vi "GetRollingAverage.vi"(8 "Error In":errorcluster, 10 "Datum":dbl, 11 "Rolling Average Queue In":refnum<queue>) -> (0 "Error Out":errorcluster, 1 "Non-Zero Rolling Average":dbl, 2 "Rolling Average":dbl format="%0.2f", 3 "Rolling Average Queue Out":refnum<queue>)   [LabVIEW 2012, in "LV-Utilities.lvlib"]
uses:
  LV-Utilities.lvlib
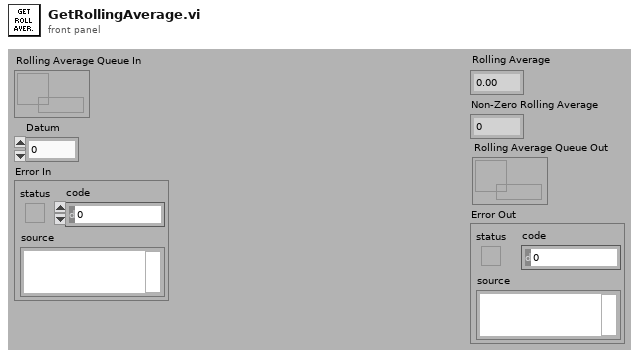
[diagram p1: front panel]
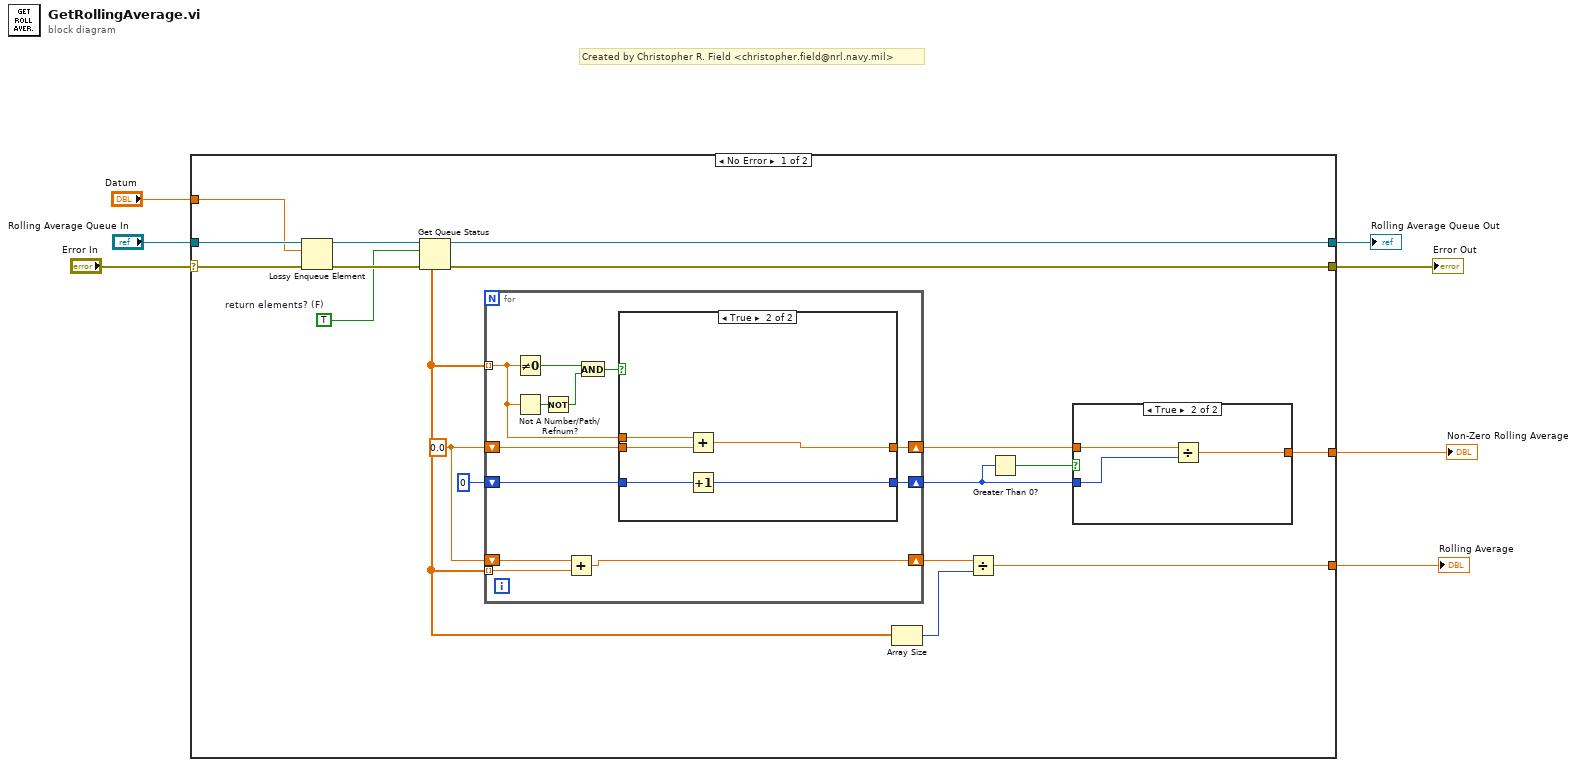
[diagram p0: block diagram]
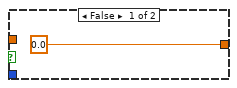
[diagram p2: hidden frame]
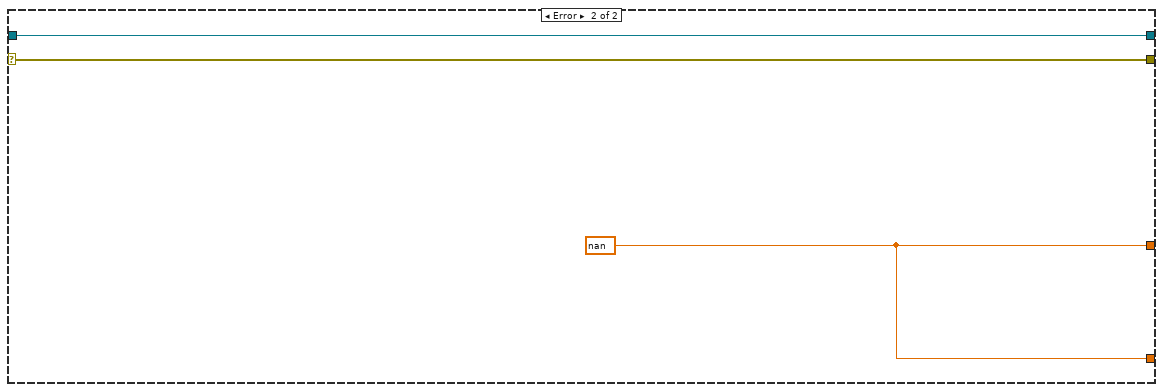
[diagram p4: hidden frame]
diagram:
  # "Created by Christopher R. Field <christopher.field@nrl.navy.mil>"
  n1 = case shown="No Error" "Error In" {
    selector: "Error In" -> [w8 w50]
    tunnel: "Rolling Average Queue In" -> [w25 w51]
    tunnel: "Datum" -> [w24 _]
    tunnel: [w18 w49] -> w5
    tunnel: [w17 w51] -> w4
    tunnel: [w16 w50] -> w3
    tunnel: [w9 w49] -> w2
    frame No Error {
      w13 = 0.0
      w21 = TRUE  # return elements? (F)
      n2 = Lossy Enqueue Element(queue=w25, element=w24, error in (no error)=w8) -> (queue out=w23:refnum<queue>, error out=w22:errorcluster)  [unwired: 2 out]
      n3 = Get Queue Status(queue=w23, return elements? (F)=w21, error in (no error)=w22) -> (queue out=w17:refnum<queue>, error out=w16:errorcluster, elements=w12:dbl[])  [unwired: 5 out]
      n4 = for {
        tunnel: w12 -> [w34] mode=indexing
        shift-right: [w38] -> w19
        shift-left: w13 -> [w41]
        shift-right: [w39] -> w15
        shift-left: 0 -> [w40]
        tunnel: w12 -> [w36] mode=indexing
        shift-right: [w35] -> w11
        shift-left: w13 -> [w37]
        n5 = Not Equal To 0?(x=w34) -> (x != 0?=w32:bool)
        n6 = Not A Number/Path/Refnum?(number/path/refnum=w34) -> (NaN/Path/Refnum?=w33:bool)
        n7 = Not(x=w33) -> (.not. x?=w31:bool)
        n8 = Add(x=w37, y=w36) -> (x+y=w35:dbl)
        n9 = And(x=w32, y=w31) -> (x .and. y?=w30:bool)
        n10 = case shown="True" w30 {
          tunnel: w34 -> [_ w48]
          tunnel: w41 -> [w43 w47]
          tunnel: w40 -> [w42 w46]
          tunnel: [w42 w45] -> w39
          tunnel: [w43 w44] -> w38
          frame False {
          }
          frame True {
            n11 = Add(x=w48, y=w47) -> (x+y=w44:dbl)
            n12 = Increment(x=w46) -> (x+1=w45:i32)
          }
        }
      }
      n13 = Array Size(array=w12) -> (size(s)=w10:i32)
      n14 = Divide(x=w11, y=w10) -> (x/y=w9:dbl)
      n15 = Greater Than 0?(x=w15) -> (x > 0?=w14:bool)
      n16 = case shown="True" w14 {
        tunnel: w19 -> [_ w29]
        tunnel: w15 -> [_ w28]
        tunnel: [0.0 w27] -> w18
        frame False {
        }
        frame True {
          n17 = Divide(x=w29, y=w28) -> (x/y=w27:dbl)
        }
      }
    }
    frame Error {
      w49 = nan
    }
  }
  "Rolling Average" <- w2
  "Non-Zero Rolling Average" <- w5
  "Rolling Average Queue Out" <- w4
  "Error Out" <- w3
